vi "plot_context_menu.vi"(10 "MenuSelection":string, 11 "Tree":refnum<vi>) -> ()   [LabVIEW 2019]
panel:
  out "Blue":u32
  # "*******************************************************************\nBiogas Plant Control\n\nAuthor: Paul Zügel\nGCSC-Frankfurt am Main 2020\n\n*******************************************************************"
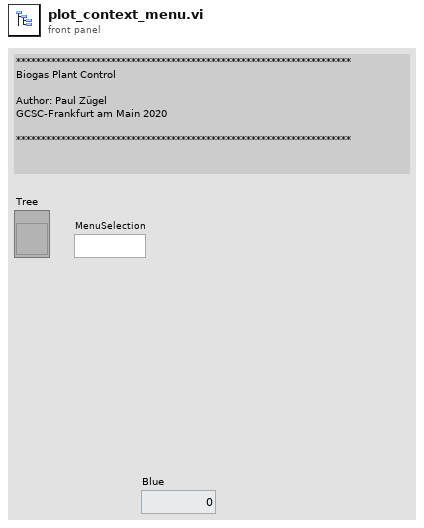
[diagram p1: front panel]
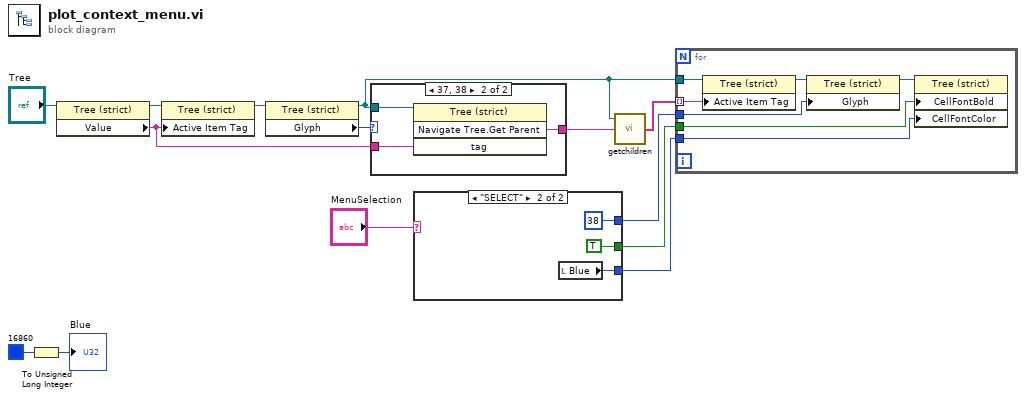
[diagram p0: block diagram]
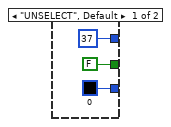
[diagram p2: hidden frame]
diagram:
  n1 = To Unsigned Long Integer(number=u32 16860) -> (unsigned 32bit integer=→"Blue":u32)
  n2 = property on="Property Node" class="Tree (strict)"(reference="Tree") -> (reference out=w14:refnum<vi>, "Value"=w3:string)  [unwired: 1 in, 1 out]
  n3 = property on="Property Node" class="Tree (strict)"(reference=w14, "Active Item Tag"=w3) -> (reference out=w13:refnum<vi>)  [unwired: 1 in, 1 out]
  n4 = property on="Property Node" class="Tree (strict)"(reference=w13) -> (reference out=w2:refnum<vi>, "Glyph"=w11:i32)  [unwired: 1 in, 1 out]
  n5 = case shown="37, 38" w11 {
    tunnel: w3 -> [w15 w17]
    tunnel: w2 -> [_ w18]
    tunnel: [w15 w16] -> w1
    frame 15, Default {
    }
    frame 37, 38 {
      n6 = invoke class="Tree (strict)" method="Navigate Tree.Get Parent"(reference=w18, "tag"=w17) -> ("Navigate Tree:Get Parent"=w16:string)  [unwired: 2 in, 3 out]
    }
  }
  n7 = case shown="\"SELECT\"" "MenuSelection" {
    tunnel: [37 ("Active Item:Symbol Index") 38 ("Active Item:Symbol Index")] -> w6
    tunnel: [FALSE ("Active Cell:Cell Font:Bold") TRUE ("Active Cell:Cell Font:Bold")] -> w7
    tunnel: [u32 0 ("Active Cell:Cell Font:Color") w22] -> w8
    frame "UNSELECT", Default {
    }
    frame "SELECT" {
      n8 = local read "Blue"() -> (w22:u32)
    }
  }
  n9 = call "getchildren.vi"("Parent Tag"=w1, "Tree Reference In"=w2) -> ("Children Tags"=w5:string[])  [unwired: 1 in, 2 out]
  n10 = for {
    tunnel: w5 -> [w30] mode=indexing
    tunnel: w2 -> [w29]
    tunnel: w6 -> [w28]
    tunnel: w7 -> [w26]
    tunnel: w8 -> [w25]
    n11 = property on="Property Node" class="Tree (strict)"(reference=w29, "Active Item Tag"=w30) -> (reference out=w31:refnum<vi>)  [unwired: 1 in, 1 out]
    n12 = property on="Property Node" class="Tree (strict)"(reference=w31, "Glyph"=w28) -> (reference out=w27:refnum<vi>)  [unwired: 1 in, 1 out]
    n13 = property class="Tree (strict)"(reference=w27, "CellFontBold"=w26, "CellFontColor"=w25) -> ()  [unwired: 1 in, 2 out]
  }
